vi "set_context_menu.vi"(8 "error in (no error)":errorcluster, 10 "Context Menu":string[][](array[string]), 11 "BalloonNotifier in":refnum<class "BalloonNotifier.lvclass">) -> (0 "error out":errorcluster, 3 "BalloonNotifier out":refnum<class "BalloonNotifier.lvclass">)   [LabVIEW 2017, in "BalloonNotifier.lvclass"]
uses:
  BalloonNotifier.lvclass
  BalloonNotifier.lvclass/BalloonNotifier.ctl
  System.Windows.Forms
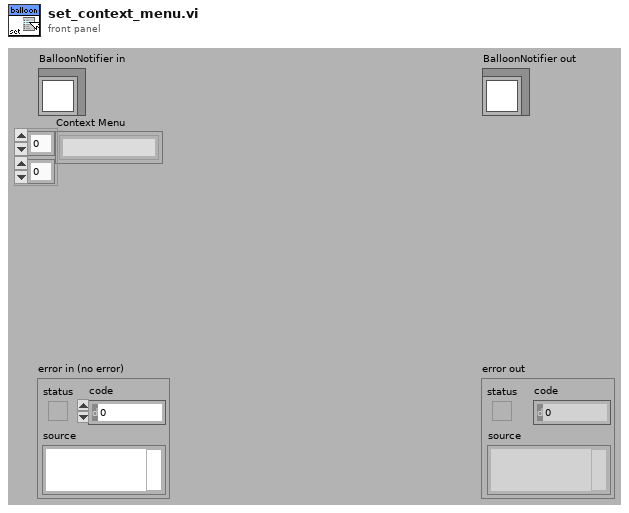
[diagram p1: front panel]
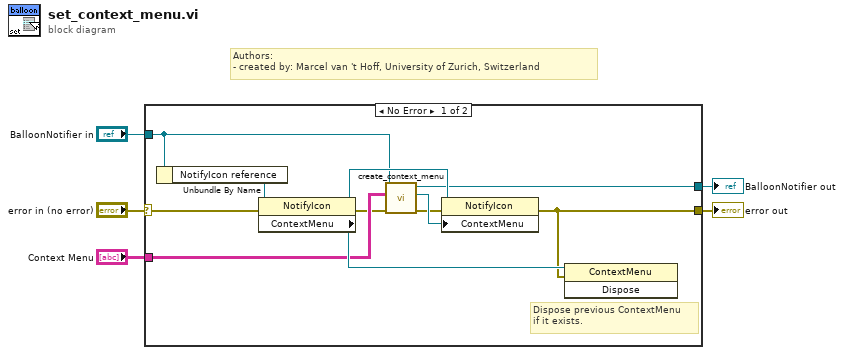
[diagram p0: block diagram]
diagram:
  # "Authors: \n- created by: Marcel van 't Hoff, University of Zurich, Switzerland"
  n1 = case shown="No Error" "error in (no error)" {
    selector: "error in (no error)" -> [w13 w18]
    tunnel: [w14 w18] -> w4
    tunnel: "Context Menu" -> [w9 _]
    tunnel: "BalloonNotifier in" -> [w11 w17]
    tunnel: [w10 w17] -> w1
    frame No Error {
      # "Dispose previous ContextMenu\nif it exists."
      n2 = Unbundle By Name(w11) -> ("NotifyIcon reference"=w12:refnum<k24>)
      n3 = property class="NotifyIcon"(reference=w12, error in=w13) -> (reference out=w16:refnum<k24>, error out=w8:errorcluster, "ContextMenu"=w15:refnum<k24>)
      n4 = call-dynamic "create_context_menu.vi"("error in (no error)"=w8, "Menus"=w9, "BalloonNotifier in"=w11) -> ("error out"=w6:errorcluster, "context menu reference"=w7:refnum<k24>, "BalloonNotifier out"=w10:refnum<class "BalloonNotifier.lvclass">)  [unwired: 6 in]
      n5 = property class="NotifyIcon"(reference=w16, error in=w6, "ContextMenu"=w7) -> (error out=w14:errorcluster)  [unwired: 1 out]
      n6 = invoke class="ContextMenu" method="Dispose"(reference=w15, error in=w14) -> ()  [unwired: 1 in, 3 out]
    }
    frame Error {
    }
  }
  "error out" <- w4
  "BalloonNotifier out" <- w1
